vi "TestPlayer.vi"(8 "error in":errorcluster, 9 "Player Color":T1, 10 "Possible Moves":bool[][](array[boolean]), 11 "Board":T3[][](array[typedef])) -> (0 "error out":errorcluster, 3 "Choice Coordinates":T2)   [LabVIEW 2020]
uses:
  Reversi/Space Ring.ctl
  Reversi/Space Coordinates.ctl
  Reversi/Turn Enum.ctl
  Reversi/Reversi.lvclass
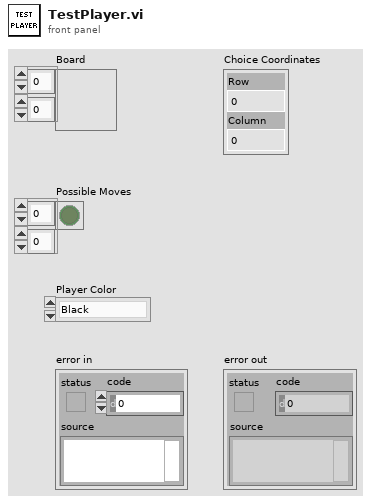
[diagram p1: front panel]
types:
  T1 = typedef "Reversi.lvlib/Reversi.lvclass/Turn Enum.ctl" = enum16{"Black", "White"}
  T2 = typedef "Reversi.lvlib/Reversi.lvclass/Space Coordinates.ctl" = cluster{"Row":i32, "Column":i32}
  T3 = typedef "Reversi.lvlib/Reversi.lvclass/Space Ring.ctl" = u16
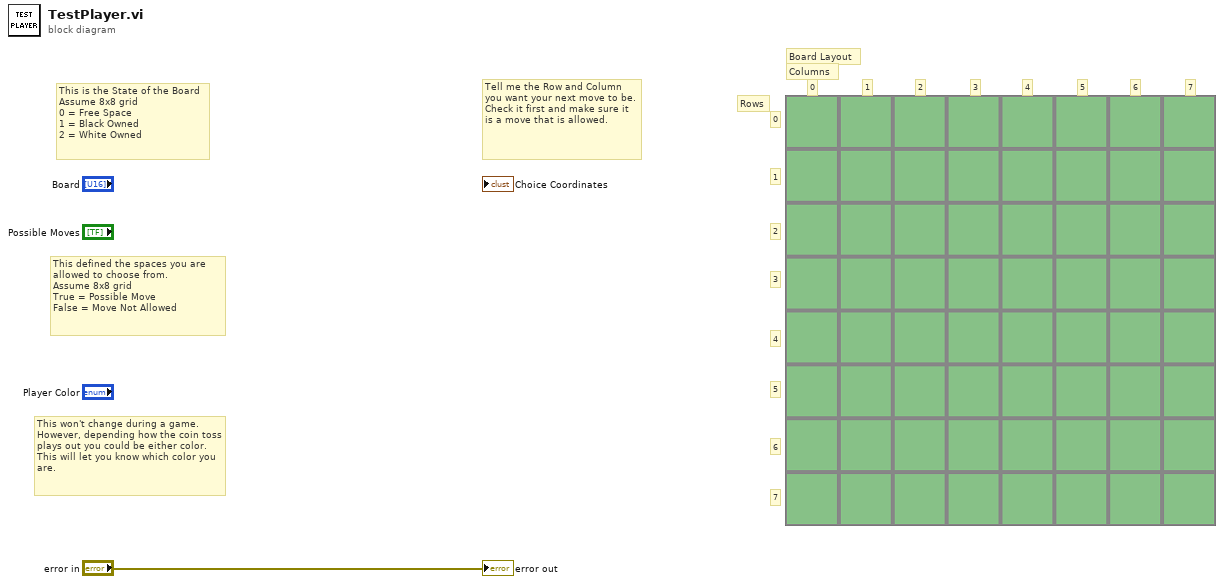
[diagram p0: block diagram]
diagram:
  # "This won't change during a game. However, depending how the coin toss plays out you could be either color. This will let you know which color you are."
  # "7"
  # "6"
  # "5"
  # "4"
  # "3"
  # "2"
  # "1"
  # "0"
  # "Rows"
  # "7"
  # "6"
  # "5"
  # "4"
  # "3"
  # "2"
  # "1"
  # "0"
  # "Columns"
  # "Board Layout"
  # "Tell me the Row and Column you want your next move to be. Check it first and make sure it is a move that is allowed."
  # "This defined the spaces you are allowed to choose from.\nAssume 8x8 grid\nTrue = Possible Move\nFalse = Move Not Allowed"
  # "This is the State of the Board\nAssume 8x8 grid\n0 = Free Space\n1 = Black Owned\n2 = White Owned"
  "error out" <- "error in"
